vi "b2-4ac.vi"(1 "C":dbl, 2 "B":dbl, 3 "A":dbl) -> (0 "b2-4ac":dbl)   [LabVIEW 2018]
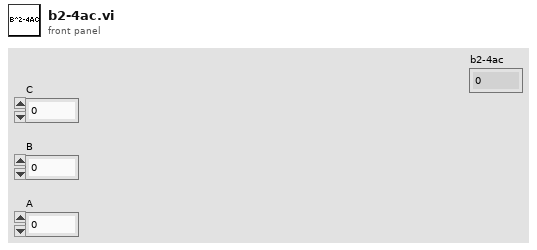
[diagram p1: front panel]
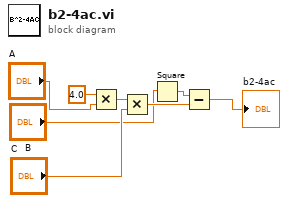
[diagram p0: block diagram]
diagram:
  n1 = Multiply(x=4.0, y="A") -> (x*y=w5:dbl)
  n2 = Multiply(x=w5, y="C") -> (x*y=w8:dbl)
  n3 = Square(x="B") -> (x^2=w7:dbl)
  n4 = Subtract(x=w7, y=w8) -> (x-y=→"b2-4ac":dbl)
